vi "Timeout.vi"(8 "error in (no error)":errorcluster, 11 "Automation Controller in":refnum<class "Automation Controller.lvclass">) -> (0 "error out":errorcluster, 3 "State Machine Actor out":refnum<class "State Machine Actor.lvclass">)   [LabVIEW 2024]
uses:
  Automation Controller.lvclass
  State Machine Actor/State Machine Actor/State Machine Actor.lvclass
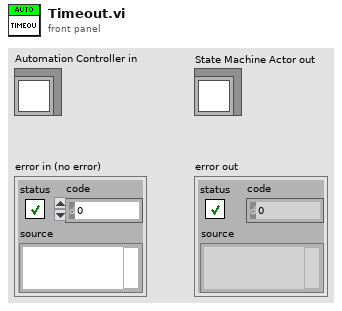
[diagram p1: front panel]
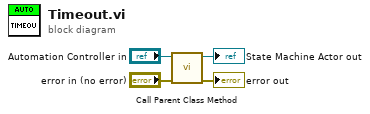
[diagram p0: block diagram]
diagram:
  n1 = call-parent "Call Parent Class Method"("error in (no error)"="error in (no error)", "State Machine Actor in"="Automation Controller in") -> ("error out"=→"error out":errorcluster, "State Machine Actor out"=→"State Machine Actor out":refnum<class "State Machine Actor.lvclass">)  [unwired: 8 in]
